vi "zc_ly.vi"(0 "action":string, 1 "LabVIEW Web Service Request":refnum<class "Web Request.lvclass"> caption="LabVIEW Web服务请求", 2 "yongtu":string, 3 "sp_yijian":string, 5 "id":string, 7 "zc_luodi_num":string, 9 "didian":string, 11 "sp_shuoming":string, 13 "shuoming":string, 14 "lc_num":string, 15 "key":string) -> (6 "error":errorcluster)   [LabVIEW 2017]
uses:
  <vilib>/wsapi/Web Request.lvclass
panel:
  out "error out":errorcluster caption="错误输出"
  in  "error 3":errorcluster={"status"=TRUE, "code"=255, "source"="当前资产不是“入库”状态！"} caption="error"
  out "postdata":string caption="post数据"
  # "Web服务请求输入接线端用于调用“Web服务”选板的VI。除非不需要访问该选板，否则不要在连线板上删除这个输入接线端。"
  # "添加至连线板的每一个其他输入控件，在URL中对应于一个输入。如需在接线端模式输出（默认设置）下包含显示控件，则该显示控件必须与连线板相连。"
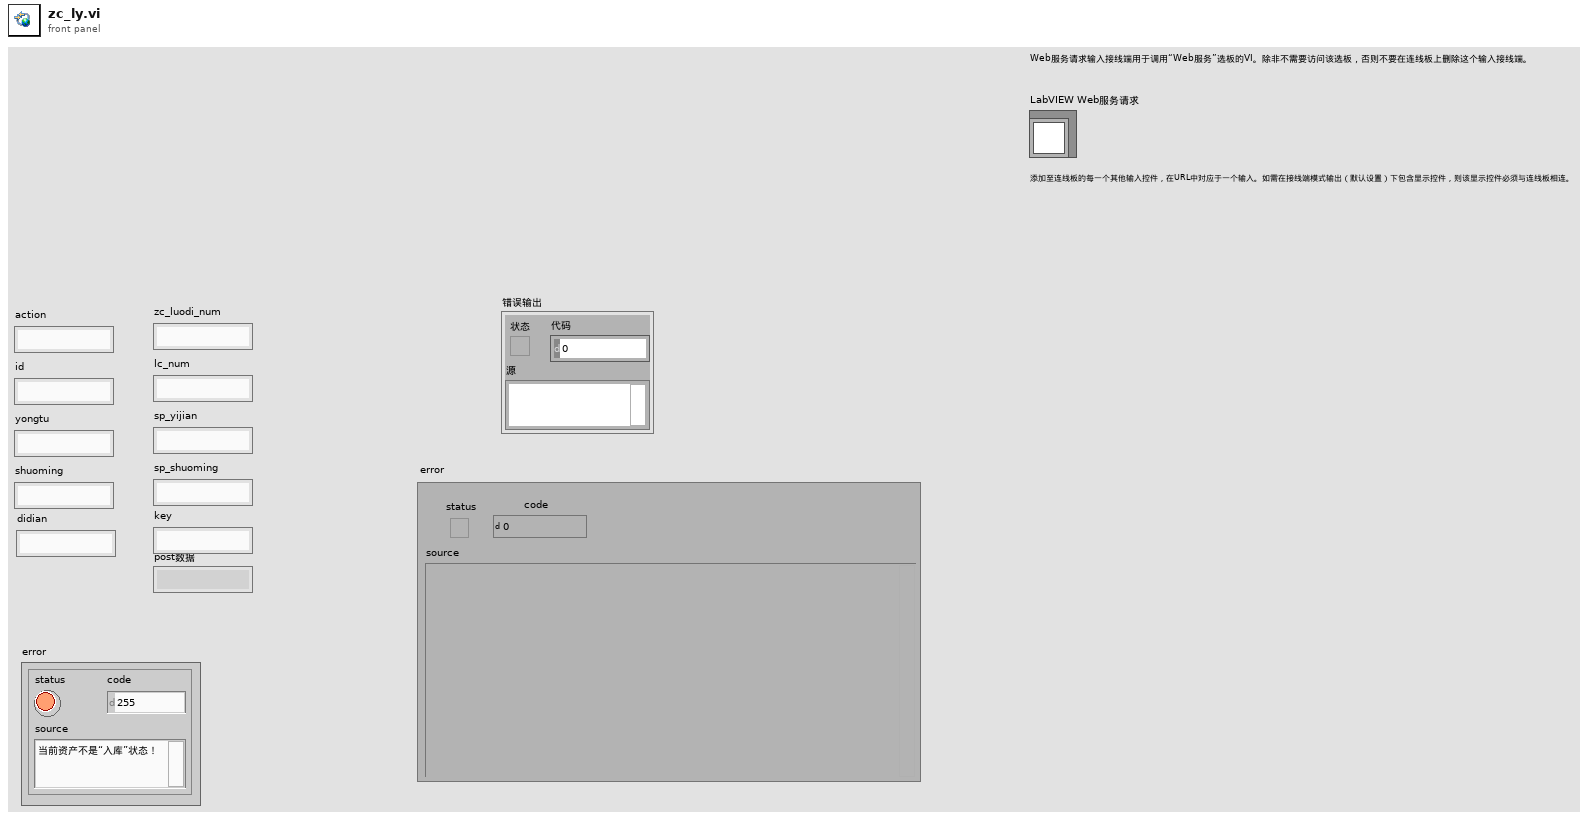
[diagram p1: front panel]
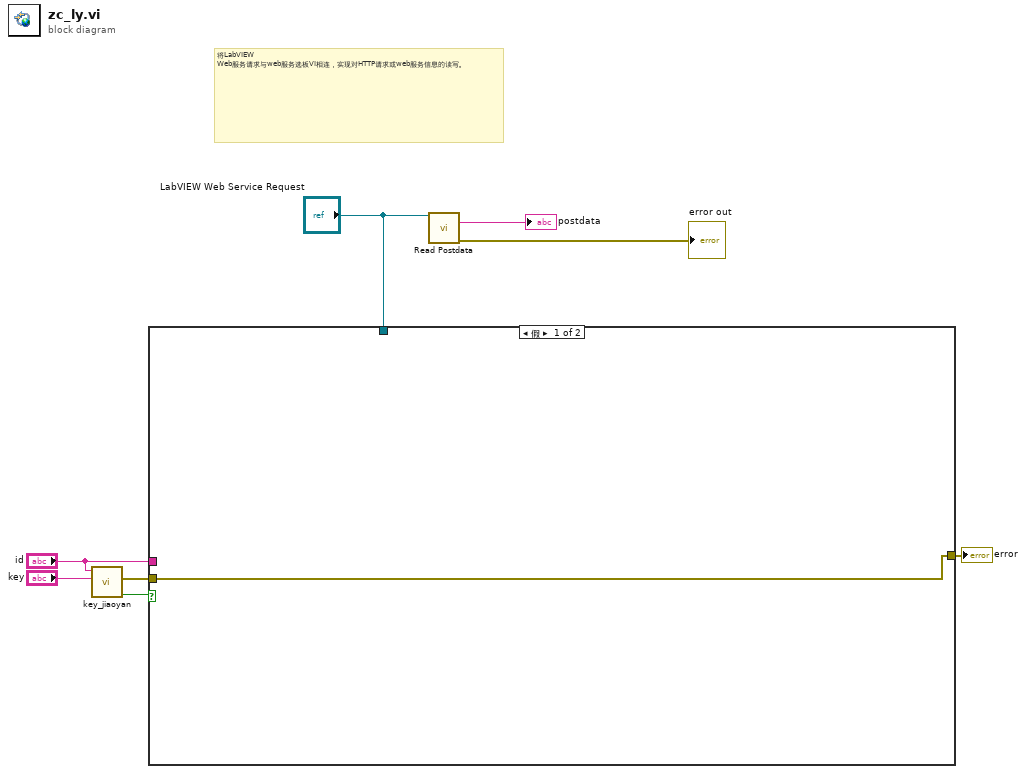
[diagram p0: block diagram]
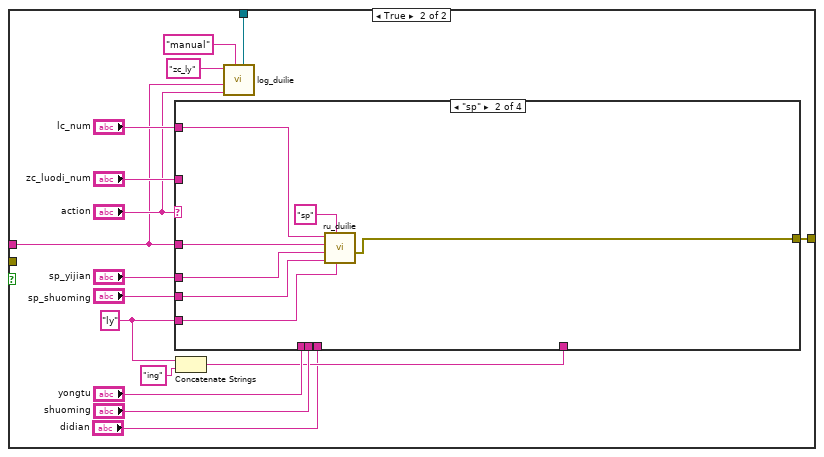
[diagram p2: hidden frame]
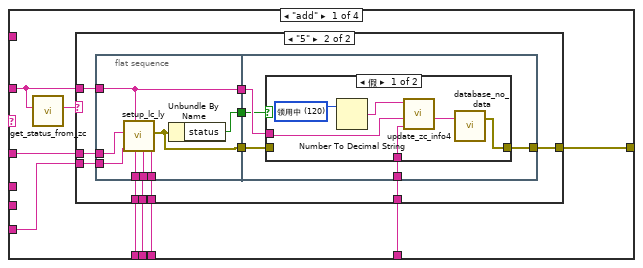
[diagram p3: hidden frame]
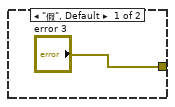
[diagram p4: hidden frame]
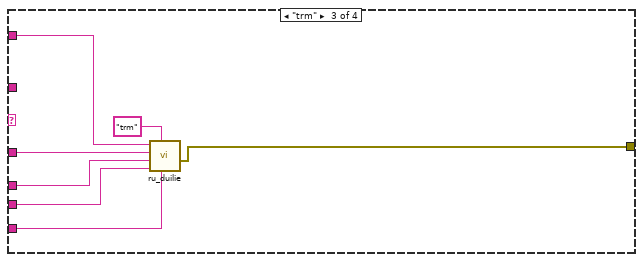
[diagram p6: hidden frame]
diagram:
  # "将LabVIEW Web服务请求与web服务选板VI相连，实现对HTTP请求或web服务信息的读写。"
  n1 = call "key_jiaoyan.vi"("key_client"="key", "gonghao"="id") -> ("jy"=w2:bool, "error"=w1:errorcluster)  [unwired: 8 in]
  n2 = case shown="假" w2 {
    tunnel: [w9 w19] -> w8
    tunnel: "LabVIEW Web Service Request" -> [_ w14]
    tunnel: "id" -> [_ w10]
    tunnel: w1 -> [w9 _]
    frame False {
    }
    frame True {
      w17 = "ly" ("yw")
      n3 = Concatenate Strings(w17, "ing" ("字符串")) -> (w16:string)
      n4 = case shown="\"sp\"" "action" {
        tunnel: w10 -> [w32 w71 w78 _]
        tunnel: "zc_luodi_num" -> [w27 _ _ _]
        tunnel: "sp_yijian" -> [_ w70 w77 _]
        tunnel: "sp_shuoming" -> [_ w69 w76 _]
        tunnel: "yongtu" -> [w34 _ _ _]
        tunnel: "shuoming" -> [w33 _ _ _]
        tunnel: w17 -> [w31 w68 w75 _]
        tunnel: "lc_num" -> [_ w72 w79 _]
        tunnel: [w30 w67 w74 _] -> w19
        tunnel: w16 -> [w29 _ _ _]
        tunnel: "didian" -> [w28 _ _ _]
        frame "add" {
          n5 = call "get_status_from_zc.vi"("zc_luodi_num"=w27) -> ("status"=w26:string)  [unwired: 9 in, 1 out]
          n6 = case shown="\"5\"" w26 {
            tunnel: w34 -> [_ w45]
            tunnel: w33 -> [_ w44]
            tunnel: w27 -> [_ w43]
            tunnel: w32 -> [_ w42]
            tunnel: w31 -> [_ w41]
            tunnel: ["error 3" w40] -> w30
            tunnel: w29 -> [_ w39]
            tunnel: w28 -> [_ w38]
            frame "假", Default {
            }
            frame "5" {
              n7 = flat-sequence {
                tunnel: w45 -> [w53]
                tunnel: w44 -> [w52]
                tunnel: w43 -> [w49]
                tunnel: w42 -> [w54]
                tunnel: w41 -> [w51]
                tunnel: [w49] -> w46
                tunnel: w38 -> [w50]
                tunnel: [w48] -> w37
                tunnel: [w47] -> w36
                tunnel: w46 -> [w58]
                tunnel: [w59] -> w40
                tunnel: w39 -> [w57]
                tunnel: w37 -> [w56]
                tunnel: w36 -> [w55]
                frame #0 {
                  n8 = call "setup_lc_ly.vi"("didian"=w50, "shuoming"=w52, "yongtu"=w53, "zc_luodi_num"=w49, "yw"=w51, "id"=w54) -> ("error"=w47:errorcluster)  [unwired: 5 in]
                  n9 = Unbundle By Name(w47) -> ("status"=w48:bool)
                }
                frame #1 {
                  n10 = case shown="假" w56 {
                    tunnel: [w63 w66] -> w59
                    tunnel: w58 -> [w62 _]
                    tunnel: w57 -> [w61 _]
                    tunnel: w55 -> [_ w66]
                    frame False {
                      w65 = u8 120 items=["待验收"=1, "无需验收"=2, "验收不合格"=3, "待入库"=4, "入库"=5, "领用"=6, "借用"=7, "托管"=8, "接管"=9, "退出"=10, "出库在用"=11, "盘亏"=12, "出售"=13, "报废"=14, "领用中"=120, "退库中"=121, "借用中"=122, "归还中"=123, "转移中"=124, "调拨中"=125, "借调中"=126, "托管中"=127, "终止托管中"=128, "退出中"=129, "处置中"=130] ("状态选择器")
                      n11 = Number To Decimal String(number=w65) -> (decimal integer string=w60:string)  [unwired: 1 in]
                      n12 = call "update_zc_info4.vi"("ywxinxi"=w61, "number"=w62, "status"=w60) -> ("data_str"=w64:string)  [unwired: 8 in]
                      n13 = call "database_no_data.vi"("input"=w64) -> ("error"=w63:errorcluster)  [unwired: 2 in]
                    }
                    frame True {
                    }
                  }
                }
              }
            }
          }
        }
        frame "sp" {
          n14 = call "ru_duilie.vi"("yw"=w68, "name"="sp" ("元素"), "sp_shuoming"=w69, "sp_yijian"=w70, "id"=w71, "lc_num"=w72) -> ("error"=w67:errorcluster)  [unwired: 5 in]
        }
        frame "trm" {
          n15 = call "ru_duilie.vi"("yw"=w75, "name"="trm" ("元素"), "sp_shuoming"=w76, "sp_yijian"=w77, "id"=w78, "lc_num"=w79) -> ("error"=w74:errorcluster)  [unwired: 5 in]
        }
        frame Default {
        }
      }
      n16 = call "log_duilie.vi"("LabVIEW Web Service Request"=w14, "type"="manual", "action"="action", "user"=w10, "yw"="zc_ly") -> ()  [unwired: 7 in]
    }
  }
  "error" <- w8
  n17 = call <vilib>:"Read Postdata.vi"("LabVIEW Web Service Request"="LabVIEW Web Service Request") -> ("postdata"=→"postdata":string, "error out"=→"error out":errorcluster)  [unwired: 12 in, 1 out]
